vi "Global Shooter Speed.vi"() -> ()   [LabVIEW 2020]
panel:
  out "Feed Forward Speed":dbl
  out "Shooter F":dbl
  out "Shooter D":dbl
  out "Shooter I":dbl
  out "Shooter P":dbl
  out "Accelerator F":dbl
  out "Accelerator D":dbl
  out "Accelerator I":dbl
  out "Accelerator P":dbl
  out "Indexer Speed Actual":dbl
  out "Feed Target":dbl
  out "Accelerator Speed Actual":dbl
  out "Accelerator Speed Target":dbl
  out "Shooter Speed Actual":dbl
  out "Shooter Speed Target":dbl
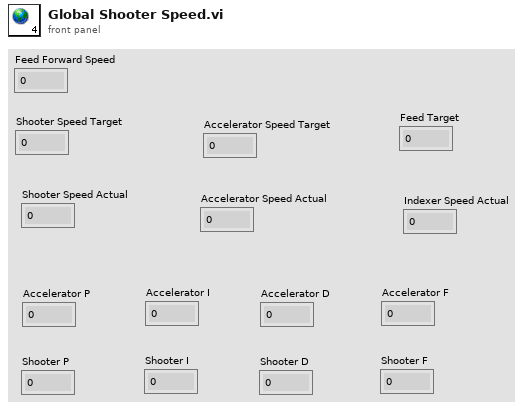
[diagram p1: front panel]
diagram:
